vi "Angulo Robo Bola.vi"(10 "Ball":T2, 11 "Robot":T1) -> (2 "Angulo":dbl)   [LabVIEW 2016]
uses:
  Core/AI Ball.ctl
  Core/AI Robot.ctl
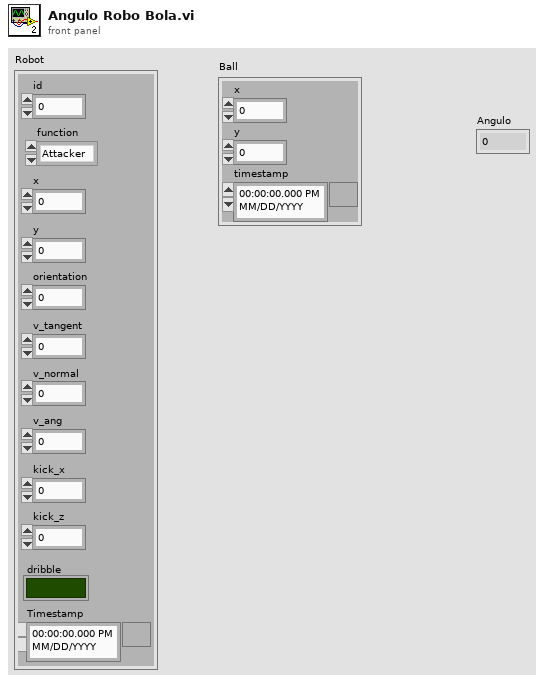
[diagram p1: front panel]
types:
  T1 = typedef "AI Robot.ctl" = cluster{"id":u32, "function":enum16{"Attacker", "Goalie", "Defender"}, "x":dbl, "y":dbl, "orientation":dbl, "v_tangent":dbl, "v_normal":dbl, "v_ang":dbl, "kick_x":dbl, "kick_z":dbl, "dribble":bool, "Timestamp":timestamp}
  T2 = typedef "AI Ball.ctl" = cluster{"x":dbl, "y":dbl, "timestamp":timestamp}
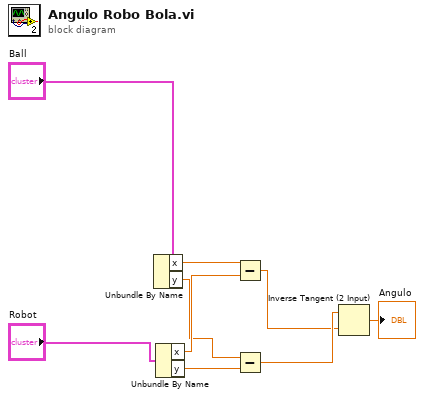
[diagram p0: block diagram]
diagram:
  n1 = Unbundle By Name("Ball") -> ("x"=w7:dbl, "y"=w5:dbl)
  n2 = Unbundle By Name("Robot") -> ("x"=w6:dbl, "y"=w4:dbl)
  n3 = Subtract(x=w7, y=w6) -> (x-y=w2:dbl)
  n4 = Subtract(x=w5, y=w4) -> (x-y=w3:dbl)
  n5 = Inverse Tangent (2 Input)(1:w2, 2:w3) -> (0:→"Angulo":dbl)
